vi "ColourUpStructures.vi"(6 "Variant in":variant, 7 "Shift Pressed?":bool, 8 "error in (no error)":errorcluster, 10 "QD Combo Box Ref":refnum<vi>, 11 "QD Launch VI Ref":refnum<vi>) -> (0 "error out":errorcluster, 4 "Variant out":variant)   [LabVIEW 2012, in "ColourUpStructures.lvlib"]
doc: "Colour Up Structures."
uses:
  ColourUpStructures.lvlib
panel:
  # "Do not change the connector pane of this VI."
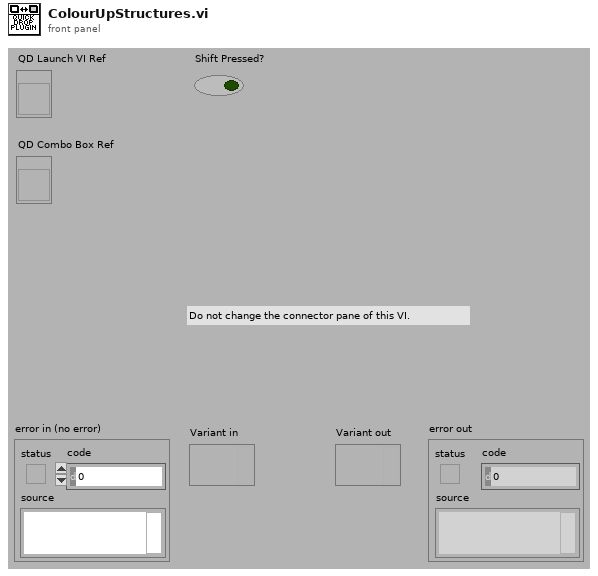
[diagram p1: front panel]
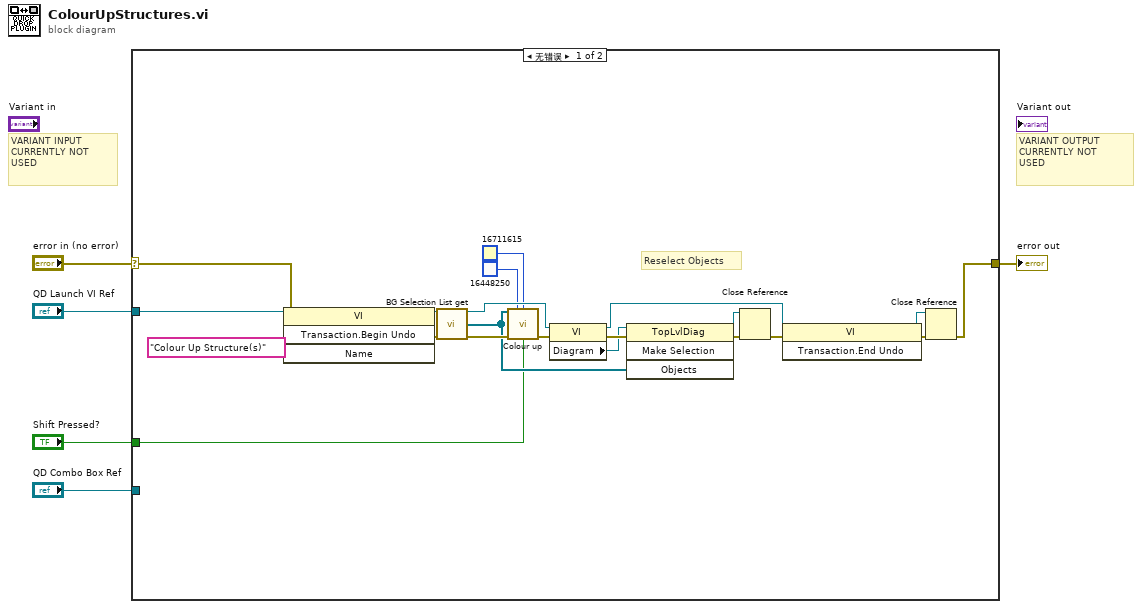
[diagram p0: block diagram]
diagram:
  # "VARIANT INPUT\nCURRENTLY NOT\nUSED"
  # "VARIANT OUTPUT\nCURRENTLY NOT\nUSED"
  n1 = case shown="无错误" "error in (no error)" {
    selector: "error in (no error)" -> [w17 w27]
    tunnel: [w11 w27] -> w4
    tunnel: "QD Launch VI Ref" -> [w19 _]
    tunnel: "Shift Pressed?" -> [w6 _]
    tunnel: "QD Combo Box Ref" -> [_ _]
    frame No Error {
      # "Reselect Objects"
      n2 = invoke class="VI" method="Transaction.Begin Undo"(reference=w19, error in=w17, "Name"="Colour Up Structure(s)") -> (reference out=w18:refnum<vi>, error out=w16:errorcluster)  [unwired: 1 in, 2 out]
      n3 = call "BG Selection List get.vi"("QD Launch VI Ref"=w18, "error in (no error)"=w16) -> ("QD Launch VI Ref out"=w22:refnum<vi>, "Selection List[]"=w7:refnum<vi>[], "error out"=w21:errorcluster)  [unwired: 11 in]
      n4 = call "Colour up.vi"("GObjects[]"=w7, "Default Colour (White)"=u32 16448250, "Defined Colour (YellowLight)"=u32 16711615, "error in (no error)"=w21, "Don't run Recursive (run)"=w6) -> ("error out"=w20:errorcluster)  [unwired: 10 in]
      n5 = property class="VI"(reference=w22, error in=w20) -> (reference out=w13:refnum<vi>, error out=w26:errorcluster, "Diagram"=w25:refnum<vi>)
      n6 = invoke class="TopLvlDiag" method="Make Selection"(reference=w25, error in=w26, "Objects"=w7) -> (reference out=w23:refnum<vi>, error out=w24:errorcluster)  [unwired: 1 in, 2 out]
      n7 = Close Reference(reference=w23, error in (no error)=w24) -> (error out=w14:errorcluster)
      n8 = invoke class="VI" method="Transaction.End Undo"(reference=w13, error in=w14) -> (reference out=w12:refnum<vi>, error out=w10:errorcluster)  [unwired: 1 in, 1 out]
      n9 = Close Reference(reference=w12, error in (no error)=w10) -> (error out=w11:errorcluster)
    }
    frame Error {
    }
  }
  "error out" <- w4
